vi "Get Temps.vi"(8 "error in":errorcluster, 11 "CPC in":refnum<class "CPC.lvclass">) -> (0 "error out":errorcluster, 2 "instrT":cluster{"cond T":dbl, "sat T":dbl, "opt T":dbl}, 3 "CPC out":refnum<class "CPC.lvclass">)   [LabVIEW 2014, in "CPC.lvclass"]
doc: "Retrieve the condenser, saturator, and optics temperatures."
uses:
  CPC.lvclass
  Controls/CmdStruct.ctl
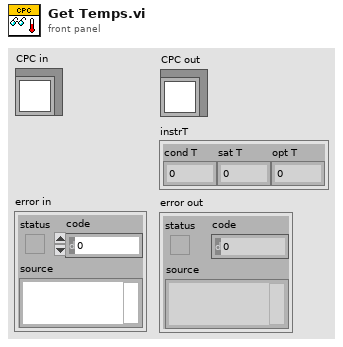
[diagram p1: front panel]
types:
  T1 = typedef "CmdStruct.ctl" = cluster{"Cmd":u8, "x":i64, "y":i64, "Display":string}
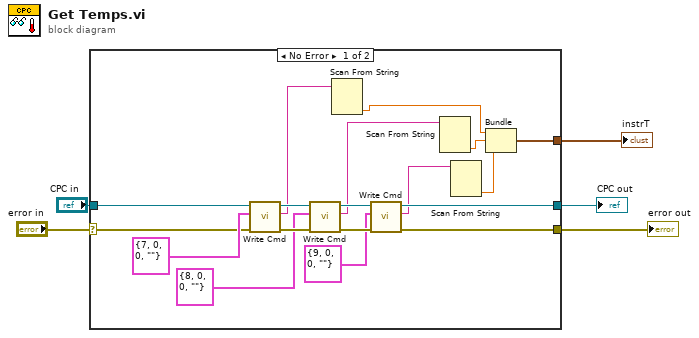
[diagram p0: block diagram]
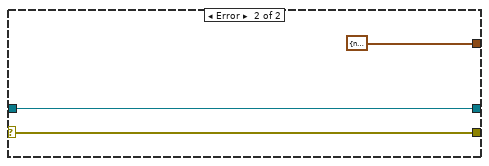
[diagram p2: hidden frame]
diagram:
  n1 = case shown="No Error" "error in" {
    selector: "error in" -> [w13 w26]
    tunnel: [w14 w26] -> w4
    tunnel: [w15 w25] -> w2
    tunnel: "CPC in" -> [w23 w25]
    tunnel: [w6 cluster{dbl, dbl, dbl} {nan, nan, nan}] -> w1
    frame No Error {
      n2 = call-dynamic "Write Cmd.vi"("error in"=w13, "CmdStruct"=T1 {"Cmd"=7, "x"=0, "y"=0, "Display"=""}, "CPC in"=w23) -> ("error out"=w20:errorcluster, "Buffer"=w12:string, "CPC out"=w21:refnum<class "CPC.lvclass">)  [unwired: 6 in]
      n3 = call-dynamic "Write Cmd.vi"("error in"=w20, "CmdStruct"=T1 {"Cmd"=8, "x"=0, "y"=0, "Display"=""}, "CPC in"=w21) -> ("error out"=w17:errorcluster, "Buffer"=w10:string, "CPC out"=w18:refnum<class "CPC.lvclass">)  [unwired: 6 in]
      n4 = Scan From String(input string=w12) -> (output 1=w11:dbl)  [unwired: 4 in, 3 out]
      n5 = call-dynamic "Write Cmd.vi"("error in"=w17, "CmdStruct"=T1 {"Cmd"=9, "x"=0, "y"=0, "Display"=""}, "CPC in"=w18) -> ("error out"=w14:errorcluster, "Buffer"=w8:string, "CPC out"=w15:refnum<class "CPC.lvclass">)  [unwired: 6 in]
      n6 = Scan From String(input string=w10) -> (output 1=w9:dbl)  [unwired: 4 in, 3 out]
      n7 = Scan From String(input string=w8) -> (output 1=w7:dbl)  [unwired: 4 in, 3 out]
      n8 = Bundle(w11, w9, w7) -> (w6:cluster{dbl, dbl, dbl})  [unwired: 1 in]
    }
    frame Error {
    }
  }
  "error out" <- w4
  "CPC out" <- w2
  "instrT" <- w1
